vi "OpenFilesInAppContext.vi"(8 "error in":errorcluster, 10 "Files to preload":path[](array[path]), 11 "Application ref in":refnum<vi>) -> (0 "error out":errorcluster, 1 "Project Refs":refnum<vi>[](array[refnum]), 2 "VI Refs":refnum<vi>[](array[refnum]), 3 "Application ref out":refnum<vi>)   [LabVIEW 2017]
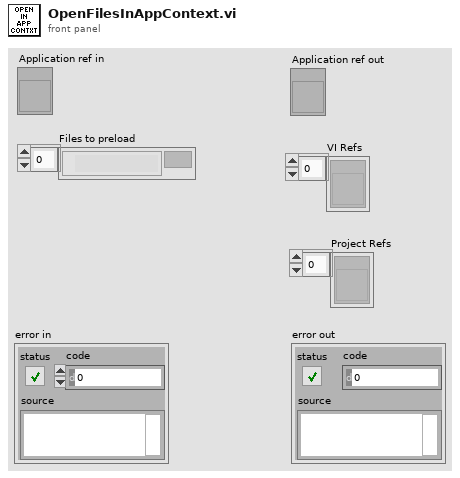
[diagram p1: front panel]
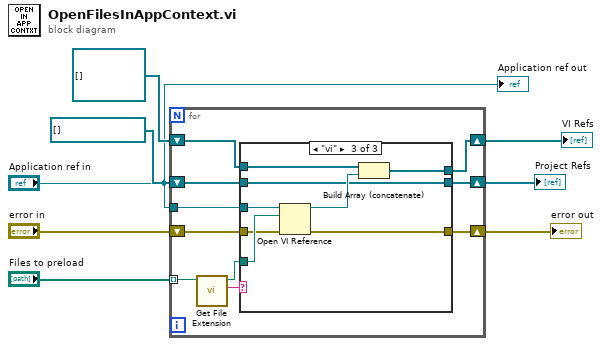
[diagram p0: block diagram]
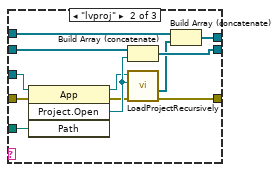
[diagram p3: hidden frame]
diagram:
  n1 = for {
    tunnel: "Files to preload" -> [w16] mode=indexing
    tunnel: "Application ref in" -> [w17]
    shift-right: [w18] -> w8
    shift-left: refnum<vi>[] [] -> [w13]
    shift-right: [w11] -> w4
    shift-left: refnum<vi>[] [] ("Project Refs 2") -> [w12]
    shift-right: [w10] -> w2
    shift-left: "error in" -> [w9]
    n2 = call <vilib>:"Get File Extension.vi"("file"=w16) -> ("lowercase file extension"=w14:string, "dup file"=w15:path)  [unwired: 6 in, 3 out]
    n3 = case shown="\"vi\"" w14 {
      tunnel: w15 -> [_ w32 w40]
      tunnel: [w20 w24 w37] -> w18
      tunnel: w17 -> [_ w33 w41]
      tunnel: [w21 w31 w36] -> w11
      tunnel: w13 -> [w20 w25 w39]
      tunnel: w12 -> [w21 w30 w36]
      tunnel: [w19 w27 w35] -> w10
      tunnel: w9 -> [w19 w23 w34]
      frame "", Default {
      }
      frame "lvproj" {
        n4 = invoke class="App" method="Project.Open"(reference=w33, error in=w23, "Path"=w32) -> (reference out=w26:refnum<vi>, error out=w28:errorcluster, "Project:Open"=w29:refnum<vi>)  [unwired: 1 in, 1 out]
        n5 = Build Array (concatenate)(w30, w29) -> (w31:refnum<vi>[])
        n6 = call "LoadProjectRecursively.vi"("error in (no error)"=w28, "Project ref in"=w29, "Application in"=w26) -> ("error out"=w27:errorcluster, "VI Refs"=w22:refnum<vi>[])  [unwired: 5 in, 2 out]
        n7 = Build Array (concatenate)(w25, w22) -> (w24:refnum<vi>[])
      }
      frame "vi" {
        n8 = Open VI Reference(application reference (local)=w41, vi path=w40, error in (no error)=w34) -> (vi reference=w38:refnum<vi>, error out=w35:errorcluster)  [unwired: 3 in]
        n9 = Build Array (concatenate)(w39, w38) -> (w37:refnum<vi>[])
      }
    }
  }
  "VI Refs" <- w8
  "Project Refs" <- w4
  "error out" <- w2
  "Application ref out" <- "Application ref in"
